vi "PH_SHS_Analysis_Statistician.ProcCases.vi"(0 "i ref in":refnum<vi>, 1 "selector":string, 2 "Data":T1, 3 "call cluster":T2={"Object"="", "Selector"="", "CallType"=enum."synchronous", "Async Object"="", "Async Selector"="", "Data Descriptor"="", "Data"=[], "Error #"=0, "Expire"=0}, 5 "error in (no error)":errorcluster) -> (14 "i ref out":refnum<vi>, 17 "answer cluster":T2={"Object"="", "Selector"="", "CallType"=enum."synchronous", "Async Object"="", "Async Selector"="", "Data Descriptor"="", "Data"=[], "Error #"=0, "Expire"=0}, 19 "error out":errorcluster)   [LabVIEW 2014, in "PH_SHS_Analysis_Statistician.lvlib"]
doc: "This method is called by a process from within the default case in the event loop. The methods of a class that are linked to events will be called from THIS method. Add your code here."
uses:
  PH_SHS_Analysis_Statistician.lvlib
  CS_Core/CSSystem/CoreDefs/CoreDefs.call_type.ctl
  CS_Core/BaseProcess/BaseProcess.descriptor string definition.ctl
  CS_Core/CSSystem/CoreDefs/CoreDefs.rawDataType.ctl
  CS_Core/CSSystem/CoreLib/CoreLib.byte array 2 short.vi
  CS_Core/CSSystem/CoreLib/CoreLib.string 2 byte array.vi
  CS_Core/CSSystem/CoreLib/CoreLib.byte array 2 int.vi
  CS_Core/CSSystem/CoreLib/CoreLib.lvlib
  CS_Core/BaseProcess/BaseProcess.lvlib
  CS_Core/CAEObj/CAEObj.lvlib
  PH_SHS_Analysis/PH_SHS_Analysis.lvlib
  PH_Basics/PH_Class/PH_Class.lvlib
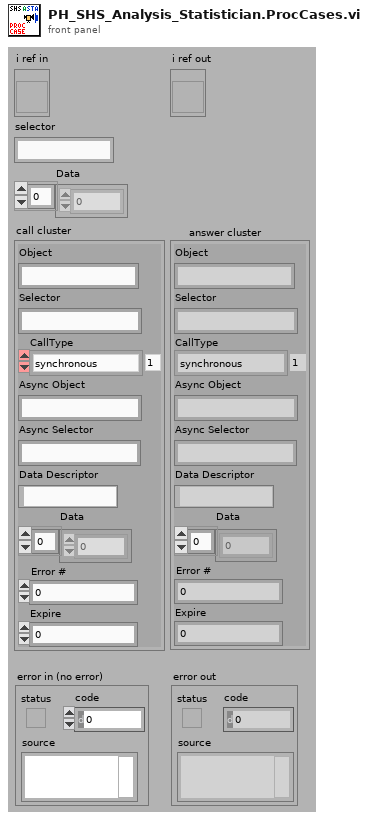
[diagram p1: front panel]
types:
  T1 = typedef "CoreDefs.rawDataType.ctl" = i8[]
  T2 = typedef "CoreDefs.call_type.ctl" = cluster{"Object":string, "Selector":string, "CallType":enum16{"simple", "synchronous", "asynchronous"}, "Async Object":string, "Async Selector":string, "Data Descriptor":T3, "Data":T1, "Error #":i32, "Expire":u32}
  T3 = typedef "BaseProcess.lvlib/BaseProcess.descriptor string definition.ctl" = string
  T4 = typedef "PH_SHS_Analysis.lvlib/PH_SHS_Analysis.Zernike Dataset.ctl" = cluster{"State":T5, "Time Stamp":timestamp, "PtV [lambda]":dbl, "Zernicke Coefficients":T6}
  T5 = typedef "PH_StatusHandler.lvlib/PH_StatusHandler.Status.ctl" = i16
  T6 = typedef "PH_SHS_Analysis.lvlib/PH_SHS_Analysis.Zernike Coefficients.ctl" = cluster{"Tilt x":dbl, "Tilt y":dbl, "Defocus":dbl, "Astig 0°":dbl, "Astig 45°":dbl, "Coma x":dbl, "Coma y":dbl, "Spherical":dbl, "Trefoil 0°":dbl, "Trefoil 30°":dbl, "2nd Astig 0°":dbl, "2nd Astig 45°":dbl, "2nd Coma x":dbl, "2nd Coma y":dbl, "2nd Spherical":dbl}
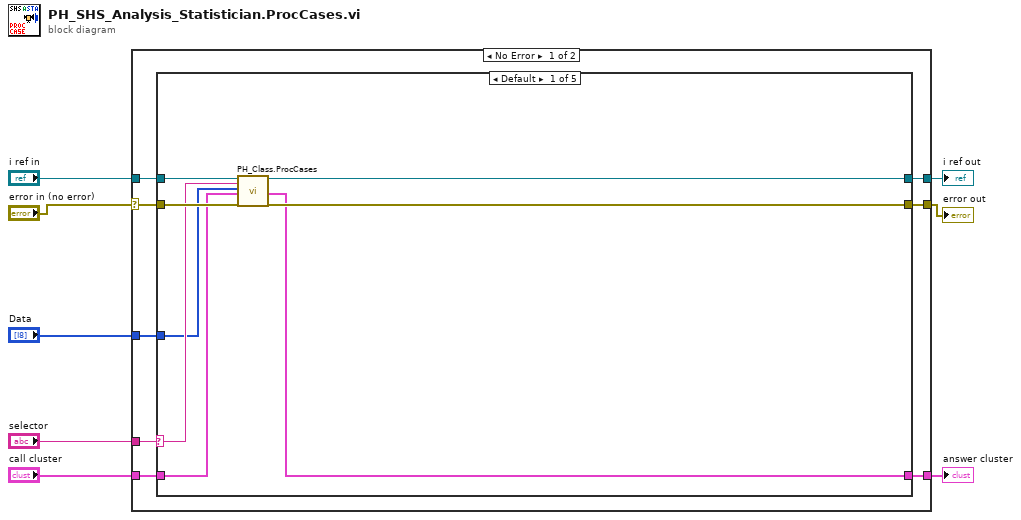
[diagram p0: block diagram]
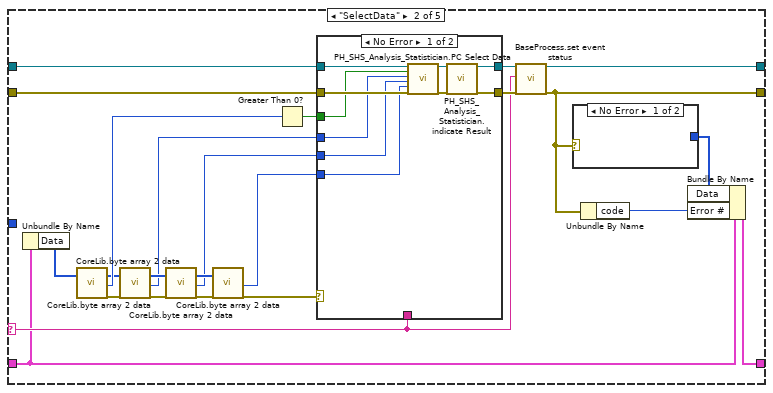
[diagram p2: hidden frame]
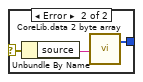
[diagram p3: hidden frame]
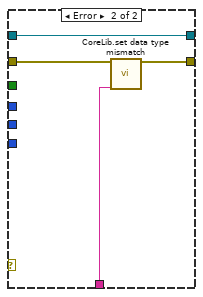
[diagram p4: hidden frame]
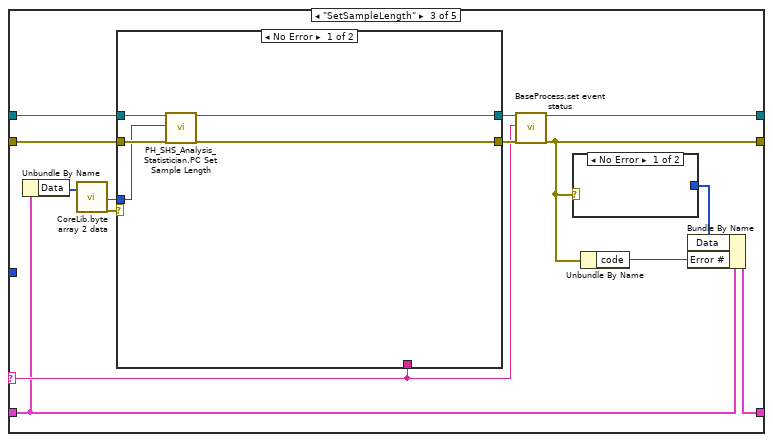
[diagram p5: hidden frame]
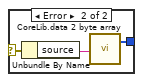
[diagram p6: hidden frame]
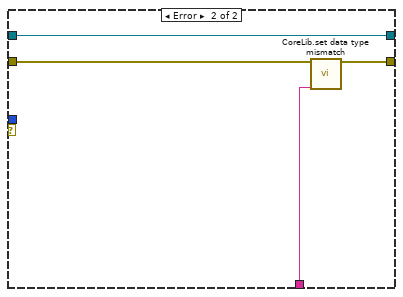
[diagram p7: hidden frame]
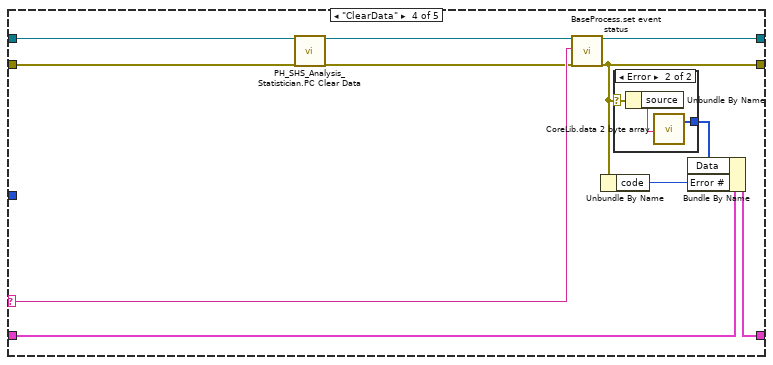
[diagram p8: hidden frame]
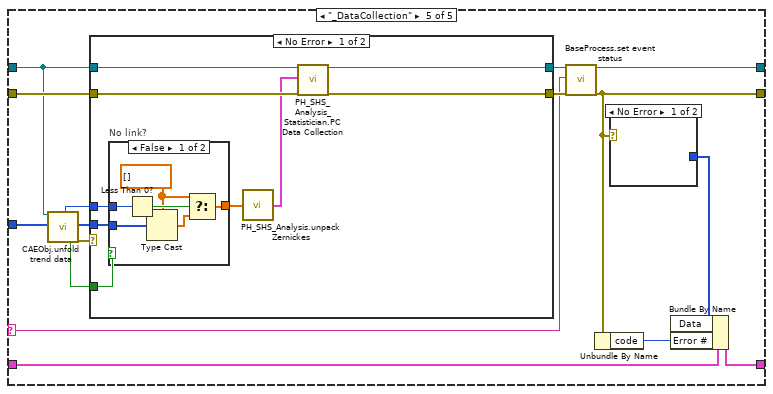
[diagram p10: hidden frame]
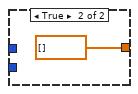
[diagram p11: hidden frame]
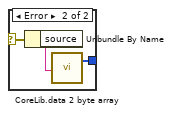
[diagram p13: hidden frame]
diagram:
  n1 = case shown="No Error" "error in (no error)" {
    selector: "error in (no error)" -> [w9 w144]
    tunnel: "selector" -> [w16 _]
    tunnel: [w15 w143] -> w7
    tunnel: "call cluster" -> [w14 w143]
    tunnel: "i ref in" -> [w13 w145]
    tunnel: [w12 w145] -> w5
    tunnel: [w11 w144] -> w4
    tunnel: "Data" -> [w10 _]
    frame No Error {
      n2 = case shown="Default" w16 {
        selector: w16 -> [w19 w37 w70 w98 w114]
        tunnel: w13 -> [w18 w41 w74 w93 w110]
        tunnel: [w24 w39 w72 w100 w116] -> w12
        tunnel: w14 -> [w20 w36 w69 w97 w113]
        tunnel: [w21 w35 w68 w96 w112] -> w15
        tunnel: w9 -> [w23 w40 w73 w95 w117]
        tunnel: [w22 w38 w71 w99 w115] -> w11
        tunnel: w10 -> [w17 _ _ _ w111]
        frame Default {
          n3 = call "PH_Class.ProcCases.vi"("i ref in"=w18, "selector"=w19, "Data"=w17, "call cluster"=w20, "error in (no error)"=w23) -> ("i ref out"=w24:refnum<vi>, "answer cluster"=w21:T2, "error out"=w22:errorcluster)  [unwired: 12 in]
        }
        frame "SelectData" {
          n4 = Unbundle By Name(w36) -> ("Data"=w44:T1)
          n5 = call-poly "CoreLib.byte array 2 data.vi"("byteArray"=w44) -> ("byteArray out"=w30:T1, "i16"=w45:i16, "error out"=w34:errorcluster)  [unwired: 16 in]
          n6 = call-poly "CoreLib.byte array 2 data.vi"("byteArray"=w30, "error in (no error)"=w34) -> ("byteArray out"=w29:T1, "i16"=w27:i16, "error out"=w33:errorcluster)  [unwired: 15 in]
          n7 = call-poly "CoreLib.byte array 2 data.vi"("byteArray"=w29, "error in (no error)"=w33) -> ("byteArray out"=w28:T1, "i16"=w26:i16, "error out"=w32:errorcluster)  [unwired: 15 in]
          n8 = call-poly "CoreLib.byte array 2 data.vi"("byteArray"=w28, "error in (no error)"=w32) -> ("i16"=w25:i16, "error out"=w31:errorcluster)  [unwired: 15 in, 1 out]
          n9 = Greater Than 0?(x=w45) -> (x > 0?=w46:bool)
          n10 = case shown="No Error" w31 {
            tunnel: [w54 w65] -> w42
            tunnel: w41 -> [w61 w65]
            tunnel: w40 -> [w60 w64]
            tunnel: [w52 w63] -> w43
            tunnel: w37 -> [_ w62]
            tunnel: w46 -> [w59 _]
            tunnel: w27 -> [w58 _]
            tunnel: w26 -> [w57 _]
            tunnel: w25 -> [w56 _]
            frame No Error {
              n11 = call "PH_SHS_Analysis_Statistician.PC Select Data.vi"("i ref in"=w61, "Stat or Trend"=w59, "Data 1"=w58, "Data 2"=w57, "Data 3"=w56, "error in (no error)"=w60) -> ("i ref out"=w55:refnum<vi>, "error out"=w53:errorcluster)  [unwired: 12 in]
              n12 = call "PH_SHS_Analysis_Statistician.indicate Result.vi"("i ref in"=w55, "error in (no error)"=w53) -> ("i ref out"=w54:refnum<vi>, "error out"=w52:errorcluster)  [unwired: 16 in]
            }
            frame Error {
              n13 = call "CoreLib.set data type mismatch.vi"("error in (no error)"=w64, "error source"=w62) -> ("error out"=w63:errorcluster)  [unwired: 17 in]
            }
          }
          n14 = call "BaseProcess.set event status.vi"("i ref in"=w42, "EventStatus"=w37, "error in (no error)"=w43) -> ("i ref out"=w39:refnum<vi>, "error out"=w38:errorcluster)  [unwired: 14 in, 1 out]
          n15 = case shown="No Error" w38 {
            selector: w38 -> [_ w51]
            tunnel: [_ w49] -> w48
            frame No Error {
            }
            frame Error {
              n16 = Unbundle By Name(w51) -> ("source"=w50:string)
              n17 = call-poly "CoreLib.data 2 byte array.vi"("string"=w50) -> ("byteArray out"=w49:T1)  [unwired: 18 in]
            }
          }
          n18 = Unbundle By Name(w38) -> ("code"=w47:i32)
          n19 = Bundle By Name(cluster=w36, "Data"=w48, "Error #"=w47) -> (w35:T2)
        }
        frame "SetSampleLength" {
          n20 = Unbundle By Name(w69) -> ("Data"=w77:T1)
          n21 = call-poly "CoreLib.byte array 2 data.vi"("byteArray"=w77) -> ("i32"=w66:i32, "error out"=w67:errorcluster)  [unwired: 16 in, 1 out]
          n22 = case shown="No Error" w67 {
            tunnel: [w85 w91] -> w75
            tunnel: w74 -> [w87 w91]
            tunnel: w73 -> [w86 w90]
            tunnel: [w84 w89] -> w76
            tunnel: w70 -> [_ w88]
            tunnel: w66 -> [w83 _]
            frame No Error {
              n23 = call "PH_SHS_Analysis_Statistician.PC Set Sample Length.vi"("i ref in"=w87, "Sample Length"=w83, "error IO"=w86) -> ("i ref out"=w85:refnum<vi>, "error out"=w84:errorcluster)  [unwired: 15 in]
            }
            frame Error {
              n24 = call "CoreLib.set data type mismatch.vi"("error in (no error)"=w90, "error source"=w88) -> ("error out"=w89:errorcluster)  [unwired: 17 in]
            }
          }
          n25 = call "BaseProcess.set event status.vi"("i ref in"=w75, "EventStatus"=w70, "error in (no error)"=w76) -> ("i ref out"=w72:refnum<vi>, "error out"=w71:errorcluster)  [unwired: 14 in, 1 out]
          n26 = case shown="No Error" w71 {
            selector: w71 -> [_ w82]
            tunnel: [_ w80] -> w79
            frame No Error {
            }
            frame Error {
              n27 = Unbundle By Name(w82) -> ("source"=w81:string)
              n28 = call-poly "CoreLib.data 2 byte array.vi"("string"=w81) -> ("byteArray out"=w80:T1)  [unwired: 18 in]
            }
          }
          n29 = Unbundle By Name(w71) -> ("code"=w78:i32)
          n30 = Bundle By Name(cluster=w69, "Data"=w79, "Error #"=w78) -> (w68:T2)
        }
        frame "ClearData" {
          n31 = call "PH_SHS_Analysis_Statistician.PC Clear Data.vi"("i ref in"=w93, "error IO"=w95) -> ("i ref out"=w92:refnum<vi>, "error out"=w94:errorcluster)  [unwired: 16 in]
          n32 = call "BaseProcess.set event status.vi"("i ref in"=w92, "EventStatus"=w98, "error in (no error)"=w94) -> ("i ref out"=w100:refnum<vi>, "error out"=w99:errorcluster)  [unwired: 14 in, 1 out]
          n33 = Unbundle By Name(w99) -> ("code"=w101:i32)
          n34 = case shown="Error" w99 {
            selector: w99 -> [_ w105]
            tunnel: [_ w103] -> w102
            frame No Error {
            }
            frame Error {
              n35 = Unbundle By Name(w105) -> ("source"=w104:string)
              n36 = call-poly "CoreLib.data 2 byte array.vi"("string"=w104) -> ("byteArray out"=w103:T1)  [unwired: 18 in]
            }
          }
          n37 = Bundle By Name(cluster=w97, "Data"=w102, "Error #"=w101) -> (w96:T2)
        }
        frame "_DataCollection" {
          n38 = call "CAEObj.unfold trend data.vi"("i ref in"=w110, "raw trend data"=w111) -> ("quality"=w107:i32, "no link"=w106:bool, "data"=w108:i8[], "error out"=w109:errorcluster)  [unwired: 9 in, 5 out]
          n39 = case shown="No Error" w109 {
            tunnel: [w130 w138] -> w119
            tunnel: [w129 w139] -> w118
            tunnel: w117 -> [w128 w138]
            tunnel: w110 -> [w126 w139]
            tunnel: w108 -> [w125 _]
            tunnel: w107 -> [w124 _]
            tunnel: w106 -> [w123 _]
            frame No Error {
              n40 = case "No link?" shown="False" w123 {
                tunnel: [w132 dbl[] []] -> w127
                tunnel: w124 -> [w136 _]
                tunnel: w125 -> [w135 _]
                frame False {
                  w131 = dbl[] []
                  n41 = Less Than 0?(x=w136) -> (x < 0?=w134:bool)
                  n42 = Type Cast(type=w131, x=w135) -> (*(type *) &x=w133:dbl[])
                  n43 = Select(t=w131, s=w134, f=w133) -> (s? t:f=w132:dbl[])
                }
                frame True {
                }
              }
              n44 = call "PH_SHS_Analysis.unpack Zernickes.vi"("DIM Service Array"=w127) -> ("SHS Analyzer Dataset"=w122:T4)
              n45 = call "PH_SHS_Analysis_Statistician.PC Data Collection.vi"("i ref in"=w126, "Data"=w122, "error IO"=w128) -> ("i ref out"=w129:refnum<vi>, "error out"=w130:errorcluster)  [unwired: 15 in]
            }
            frame Error {
            }
          }
          n46 = call "BaseProcess.set event status.vi"("i ref in"=w118, "EventStatus"=w114, "error in (no error)"=w119) -> ("i ref out"=w116:refnum<vi>, "error out"=w115:errorcluster)  [unwired: 14 in, 1 out]
          n47 = Unbundle By Name(w115) -> ("code"=w120:i32)
          n48 = case shown="No Error" w115 {
            selector: w115 -> [_ w142]
            tunnel: [_ w140] -> w121
            frame No Error {
            }
            frame Error {
              n49 = Unbundle By Name(w142) -> ("source"=w141:string)
              n50 = call-poly "CoreLib.data 2 byte array.vi"("string"=w141) -> ("byteArray out"=w140:T1)  [unwired: 18 in]
            }
          }
          n51 = Bundle By Name(cluster=w113, "Data"=w121, "Error #"=w120) -> (w112:T2)
        }
      }
    }
    frame Error {
    }
  }
  "answer cluster" <- w7
  "i ref out" <- w5
  "error out" <- w4
